vi "processData.vi"(8 "error in (no error)":errorcluster, 10 "model":refnum<class "Model.lvclass">, 11 "RampingUpPressureSTState in":refnum<class "RampingUpPressureSTState.lvclass">) -> (0 "error out":errorcluster, 2 "model 2":refnum<class "Model.lvclass">, 3 "RampingUpPressureSTState out":refnum<class "RampingUpPressureSTState.lvclass">)   [LabVIEW 2015, in "RampingUpPressureSTState.lvclass"]
uses:
  RampingUpPressureSTState.lvclass
  Model/Model/Model.lvclass
  TestingStiffnessState/TestingStiffnessState.lvclass
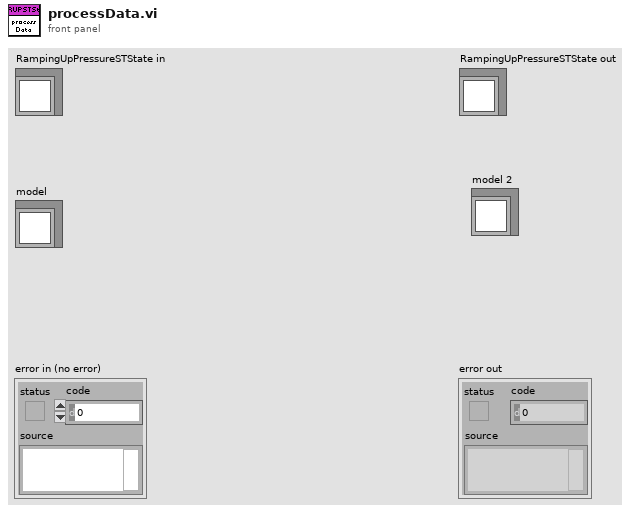
[diagram p1: front panel]
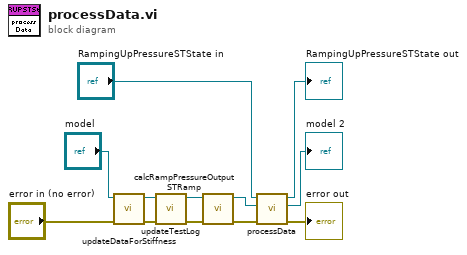
[diagram p0: block diagram]
diagram:
  n1 = call "updateDataForStiffness.vi"("error in (no error)"="error in (no error)", "Model in"="model") -> ("error out"=w1:errorcluster, "Model out"=w2:refnum<class "Model.lvclass">)  [unwired: 8 in]
  n2 = call "updateTestLog.vi"("error in (no error)"=w1, "Model in"=w2) -> ("error out"=w3:errorcluster, "Model out"=w4:refnum<class "Model.lvclass">)  [unwired: 8 in]
  n3 = call "calcRampPressureOutputSTRamp.vi"("error in (no error)"=w3, "Model in"=w4) -> ("error out"=w5:errorcluster, "Model out"=w6:refnum<class "Model.lvclass">)  [unwired: 8 in]
  n4 = call-parent "processData.vi"("error in (no error)"=w5, "model"=w6, "TestingState in"="RampingUpPressureSTState in") -> ("error out"=→"error out":errorcluster, "model 2"=→"model 2":refnum<class "Model.lvclass">, "TestingState out"=→"RampingUpPressureSTState out":refnum<class "RampingUpPressureSTState.lvclass">)  [unwired: 6 in]
